vi "solar_misc LVClass Descendants.vi"(8 "error in (no error)":errorcluster, 11 "Parent LVClass (*.lvclass)":string) -> (0 "error out":errorcluster, 3 "Descendants":string[](array[string]))   [LabVIEW 2018]
doc: "This VI gets the descendants of a parent LabVIEW Class (*.lvclass) in memory.\n\nCreated By: Ryan Pacini\nDate: 5/28/2016"
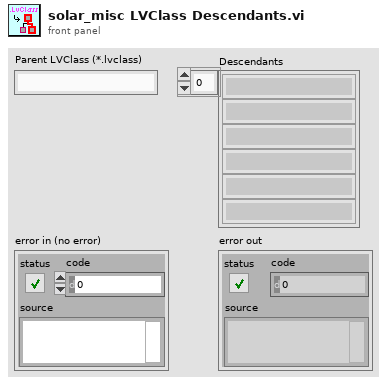
[diagram p1: front panel]
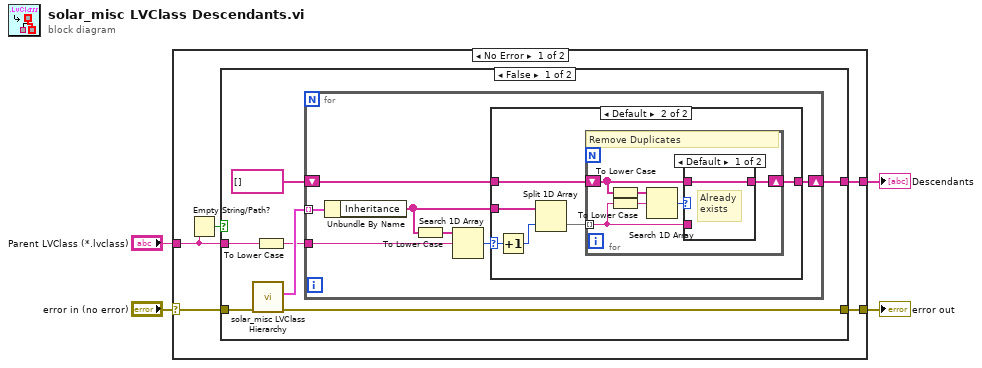
[diagram p0: block diagram]
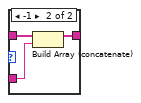
[diagram p3: hidden frame]
diagram:
  n1 = case shown="No Error" "error in (no error)" {
    selector: "error in (no error)" -> [w6 w42]
    tunnel: [w9 _] -> w4
    tunnel: "Parent LVClass (*.lvclass)" -> [w8 _]
    tunnel: [w5 w42] -> w1
    frame No Error {
      n2 = Empty String/Path?(string/path=w8) -> (empty?=w7:bool)
      n3 = case shown="False" w7 {
        tunnel: w8 -> [w14 _]
        tunnel: [w12 _] -> w9
        tunnel: w6 -> [w11 w41]
        tunnel: [w10 w41] -> w5
        frame False {
          n4 = call "solar_misc LVClass Hierarchy.vi"("error in (no error)"=w11) -> ("error out"=w10:errorcluster, "LVClass Hierarchy"=w16:cluster{"Inheritance":string[]}[])  [unwired: 8 in, 1 out]
          n5 = To Lower Case(string=w14) -> (all lower case string=w15:string)
          n6 = for {
            tunnel: w16 -> [w23] mode=indexing
            tunnel: w15 -> [w21]
            shift-right: [w17] -> w12
            shift-left: string[] [] -> [w18]
            n7 = Unbundle By Name(w23) -> ("Inheritance"=w19:string[])
            n8 = To Lower Case(string=w19) -> (all lower case string=w22:string[])
            n9 = Search 1D Array(1D array=w22, element=w21) -> (index of element=w20:i32)  [unwired: 1 in]
            n10 = case shown="Default" w20 {
              selector: w20 -> [_ w30]
              tunnel: w19 -> [_ w29]
              tunnel: w18 -> [w24 w27]
              tunnel: [w24 w26] -> w17
              frame -1 {
              }
              frame Default {
                n11 = Increment(x=w30) -> (x+1=w28:i32)
                n12 = Split 1D Array(array=w29, index=w28) -> (second subarray=w25:string[])  [unwired: 1 out]
                n13 = for {
                  shift-right: [w32] -> w26
                  shift-left: w27 -> [w33]
                  tunnel: w25 -> [w31] mode=indexing
                  # "Remove Duplicates"
                  n14 = To Lower Case(string=w33) -> (all lower case string=w36:string[])
                  n15 = To Lower Case(string=w31) -> (all lower case string=w35:string)
                  n16 = Search 1D Array(1D array=w36, element=w35) -> (index of element=w34:i32)  [unwired: 1 in]
                  n17 = case shown="Default" w34 {
                    tunnel: [w37 w40] -> w32
                    tunnel: w33 -> [w37 w39]
                    tunnel: w31 -> [_ w38]
                    frame Default {
                      # "Already\nexists"
                    }
                    frame -1 {
                      n18 = Build Array (concatenate)(w39, w38) -> (w40:string[])
                    }
                  }
                }
              }
            }
          }
        }
        frame True {
        }
      }
    }
    frame Error {
    }
  }
  "Descendants" <- w4
  "error out" <- w1
